vi "LOGIC_chkAndClearDiscardedImage.vi"(8 "error in":errorcluster) -> (0 "error out":errorcluster)   [LabVIEW 2016]
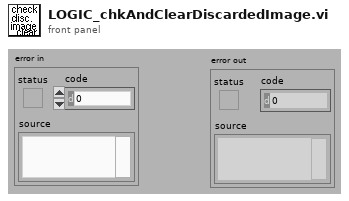
[diagram p1: front panel]
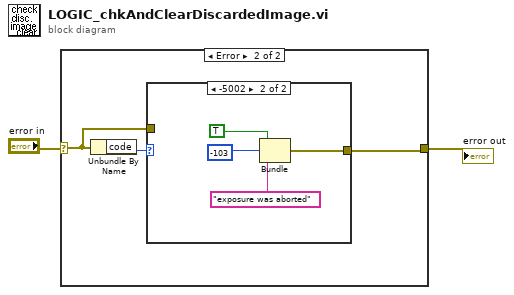
[diagram p0: block diagram]
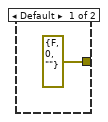
[diagram p3: hidden frame]
diagram:
  n1 = case shown="Error" "error in" {
    selector: "error in" -> [w3 w4]
    tunnel: [w3 w5] -> w1
    frame No Error {
    }
    frame Error {
      n2 = Unbundle By Name(w4) -> ("code"=w6:i32)
      n3 = case shown="-5002" w6 {
        tunnel: [errorcluster {FALSE, 0, ""} w8] -> w5
        tunnel: w4 -> [_ _]
        frame Default {
        }
        frame -5002 {
          n4 = Bundle(TRUE, -103, "exposure was aborted") -> (w8:errorcluster)  [unwired: 1 out]
        }
      }
    }
  }
  "error out" <- w1
